vi "ad sample to float64.vi"(6 "data":u64, 7 "dbl":dbl, 8 "error in (no error)":errorcluster, 9 "range":u64, 10 "cha":i32, 11 "adh":i32) -> (0 "error out":errorcluster, 3 "function return":i32, 5 "dbl out":dbl)   [LabVIEW 2021, in "libad4.lvlib"]
doc: "ad_sample_to_float64 (int32_t adh, int32_t cha, uint64_t range, uint64_t data, double *dbl);"
uses:
  <userlib>/libad4/libad4.lvlib
  <userlib>/libad4/libad4.dll
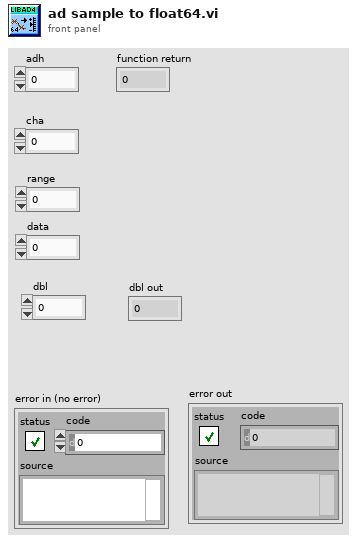
[diagram p1: front panel]
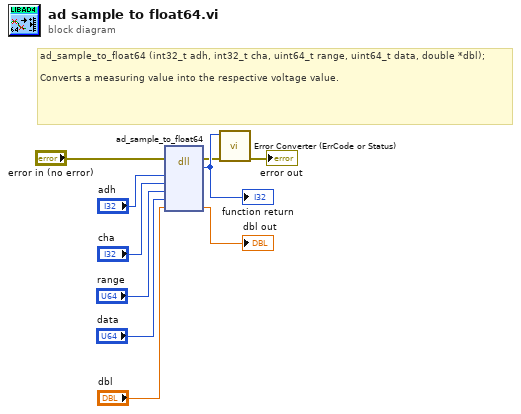
[diagram p0: block diagram]
diagram:
  # "ad_sample_to_float64 (int32_t adh, int32_t cha, uint64_t range, uint64_t data, double *dbl);\n\nConverts a measuring value into the respective voltage value."
  n1 = dll-call lib="C:/Program Files/National Instruments/LabVIEW 2021/user.lib/libad4/libad4.*" fn="ad_sample_to_float64"(error in="error in (no error)", "adh"="adh", "cha"="cha", "range"="range", "data"="data", "dbl"="dbl") -> (error out=w4:errorcluster, "return type"=w10:i32, "dbl"=→"dbl out":dbl)  [unwired: 6 in, 1 out]
  "function return" <- w10
  n2 = call <userlib>:"Error Converter (ErrCode or Status).vi"("error in (no error)"=w4, "error code"=w10) -> ("error out"=→"error out":errorcluster)  [unwired: 9 in]
